vi "Configure Temperature.vi"   [LabVIEW 2015, in "Keithley DMM6500 DAQ6500 Series.lvlib"]
doc: "Configures Temperature measurement."
uses:
  <instrlib>/Keithley DMM6500 DAQ6500 Series/Keithley DMM6500 DAQ6500 Series.lvlib
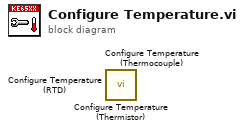
[diagram p0: block diagram]
diagram:
  n1 = call <instrlib>:"Configure Temperature (Thermistor).vi"() -> ()  [unwired: 14 in, 2 out]
  n2 = call <instrlib>:"Configure Temperature (Thermocouple).vi"() -> ()  [unwired: 14 in, 2 out]
  n3 = call <instrlib>:"Configure Temperature (RTD).vi"() -> ()  [unwired: 14 in, 2 out]
